vi "PLC.WriteValues.vi"(8 "error in":errorcluster, 10 "Slot":i32, 11 "Data_in":T1={"Status"={"Idx"=0, "ConnRef"=0, "State"=enum."Off", "LiveBitTimer"=timestamp(0 s since 1904-01-01)}, "Sets"={"Enable"=FALSE, "IP"="", "Rack"=0, "Slot"=0, "LifeBitTimer_s"=0.0, "DataBlockAddr_PCStatus"=0, "DataBlockAddr_PLCStatus"=1, "DataBlockAddr_PLCNewData"=[], "DataBlockSize_PLCNewData"=[], "DataBlockAddr_PLCChangeOver"=[], "DataBlockSize_PLCChangeOver"=[], "DataBlockAddr_PCChangeOver"=[], "DataBlockAddr_PLCCheckStatus"=[], "DataBlockSize_PLCCheckStatus"=[], "DataBlockAddr_PCCheckStatus"=[]}, "PCstatus"={"General"={"LifeBit"=FALSE, "DbRun"=FALSE}, "Stations"=[]}, "PLCstatus"={"General"={"LifeBit"=FALSE}, "Stations"=[]}}) -> (0 "error out":errorcluster, 3 "Data_out":T1={"Status"={"Idx"=0, "ConnRef"=0, "State"=enum."Off", "LiveBitTimer"=timestamp(0 s since 1904-01-01)}, "Sets"={"Enable"=FALSE, "IP"="", "Rack"=0, "Slot"=0, "LifeBitTimer_s"=0.0, "DataBlockAddr_PCStatus"=0, "DataBlockAddr_PLCStatus"=1, "DataBlockAddr_PLCNewData"=[], "DataBlockSize_PLCNewData"=[], "DataBlockAddr_PLCChangeOver"=[], "DataBlockSize_PLCChangeOver"=[], "DataBlockAddr_PCChangeOver"=[], "DataBlockAddr_PLCCheckStatus"=[], "DataBlockSize_PLCCheckStatus"=[], "DataBlockAddr_PCCheckStatus"=[]}, "PCstatus"={"General"={"LifeBit"=FALSE, "DbRun"=FALSE}, "Stations"=[]}, "PLCstatus"={"General"={"LifeBit"=FALSE}, "Stations"=[]}})   [LabVIEW 2016]
doc: "Get test results (measurement values) from PLC and save to database\n\nWabco 2017 All right reserved\nAuthor: maciej.szupienko@wabco-auto.com"
uses:
  LowLevel/PLC.DataBlock.PLCvalues.ctl
  PLC.Data.Sets.ctl
  PLC.State.ctl
  PLC.Data.Status.ctl
  PLC.Data.ctl
  LowLevel/PLC.DataBlock.PCstatus.ctl
  LowLevel/PLC.DataBlock.PLCstatus.ctl
  LowLevel/PLC.DataBlock.PLCstatus.Station.ctl
  LowLevel/PLC.DataBlock.PLCstatus.General.ctl
  LowLevel/PLC.DataBlock.PCstatus.Station.ctl
  LowLevel/PLC.DataBlock.PCstatus.General.ctl
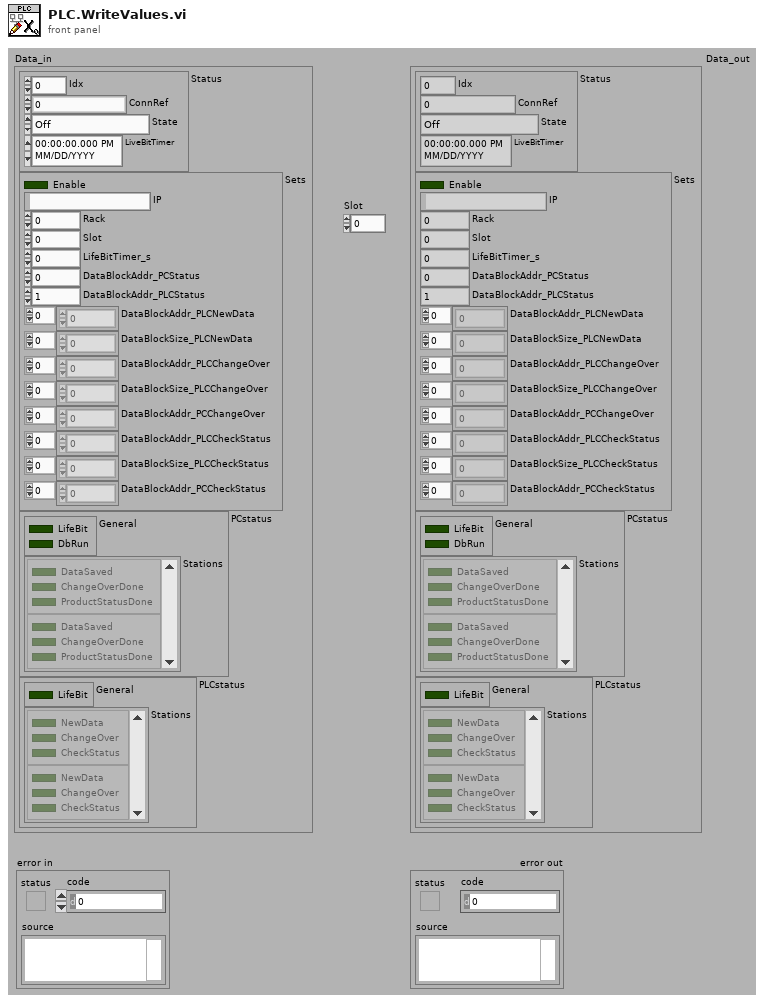
[diagram p1: front panel]
types:
  T1 = typedef "PLC.Data.ctl" = cluster{"Status":T2, "Sets":T4, "PCstatus":T5, "PLCstatus":T8}
  T2 = typedef "PLC.Data.Status.ctl" = cluster{"Idx":i32, "ConnRef":u64, "State":T3, "LiveBitTimer":timestamp}
  T3 = typedef "PLC.State.ctl" = enum32{"Off", "Error", "Idle", "Run"}
  T4 = typedef "PLC.Data.Sets.ctl" = cluster{"Enable":bool, "IP":string, "Rack":i32, "Slot":i32, "LifeBitTimer_s":dbl, "DataBlockAddr_PCStatus":i32, "DataBlockAddr_PLCStatus":i32, "DataBlockAddr_PLCNewData":i32[], "DataBlockSize_PLCNewData":i32[], "DataBlockAddr_PLCChangeOver":i32[], "DataBlockSize_PLCChangeOver":i32[], "DataBlockAddr_PCChangeOver":i32[], "DataBlockAddr_PLCCheckStatus":i32[], "DataBlockSize_PLCCheckStatus":i32[], "DataBlockAddr_PCCheckStatus":i32[]}
  T5 = typedef "PLC.DataBlock.PCstatus.ctl" = cluster{"General":T6, "Stations":T7[]}
  T6 = typedef "PLC.DataBlock.PCstatus.General.ctl" = cluster{"LifeBit":bool, "DbRun":bool}
  T7 = typedef "PLC.DataBlock.PCstatus.Station.ctl" = cluster{"DataSaved":bool, "ChangeOverDone":bool, "ProductStatusDone":bool}
  T8 = typedef "PLC.DataBlock.PLCstatus.ctl" = cluster{"General":T9, "Stations":T10[]}
  T9 = typedef "PLC.DataBlock.PLCstatus.General.ctl" = cluster{"LifeBit":bool}
  T10 = typedef "PLC.DataBlock.PLCstatus.Station.ctl" = cluster{"NewData":bool, "ChangeOver":bool, "CheckStatus":bool}
  T11 = typedef "PLC.DataBlock.PLCvalues.ctl" = cluster{"Status":u8, "Ref1":string, "Serial1":string, "Ref2":string, "Serial2":string, "Values":sgl[]}
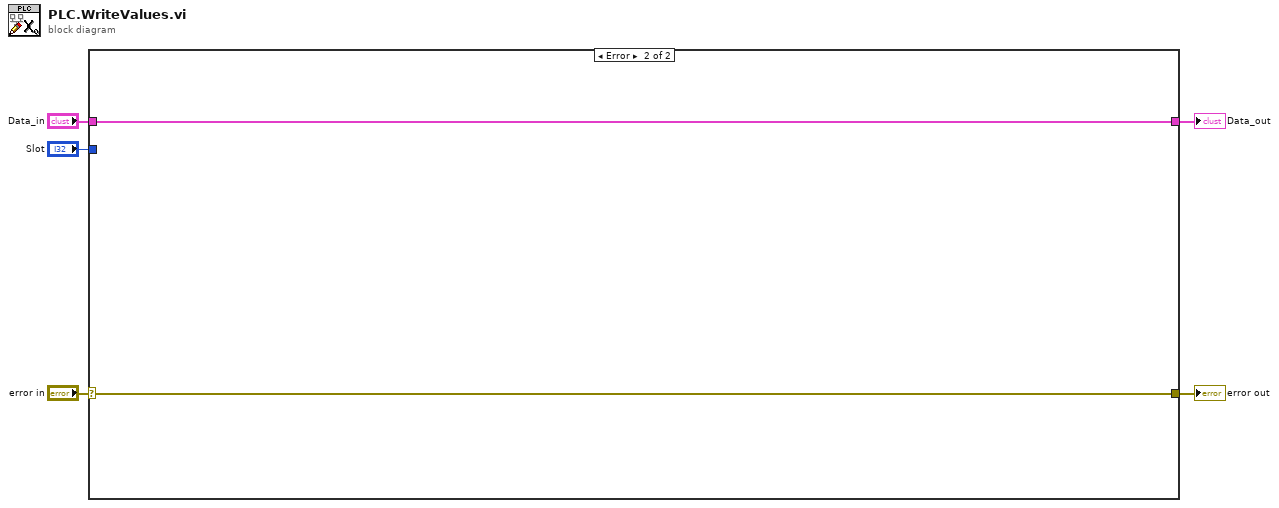
[diagram p0: block diagram]
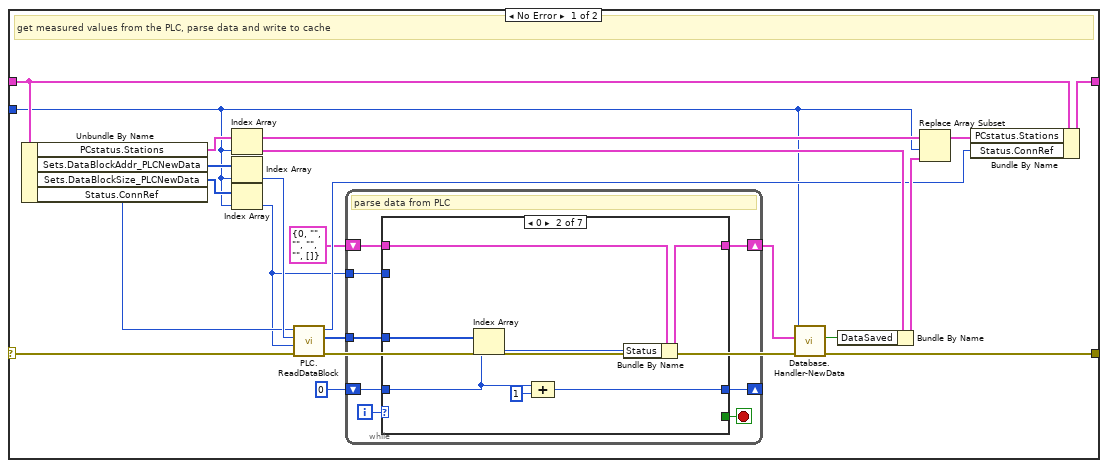
[diagram p2: hidden frame]
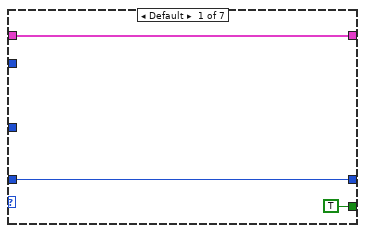
[diagram p3: hidden frame]
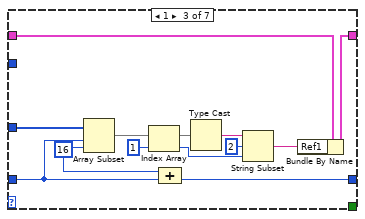
[diagram p4: hidden frame]
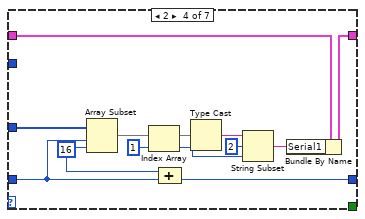
[diagram p5: hidden frame]
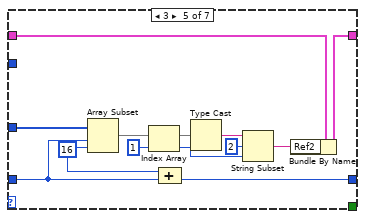
[diagram p6: hidden frame]
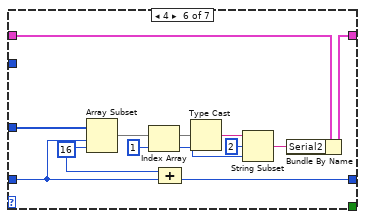
[diagram p7: hidden frame]
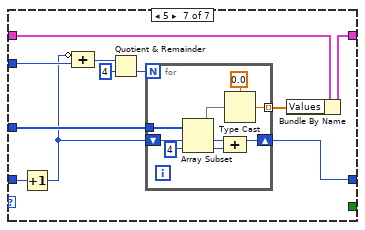
[diagram p8: hidden frame]
diagram:
  n1 = case shown="Error" "error in" {
    selector: "error in" -> [w25 w112]
    tunnel: [w6 w112] -> w2
    tunnel: "Data_in" -> [w22 w111]
    tunnel: [w26 w111] -> w4
    tunnel: "Slot" -> [w10 _]
    frame No Error {
      # "get measured values from the PLC, parse data and write to cache"
      n2 = Unbundle By Name(w22) -> ("PCstatus.Stations"=w12:T7[], "Sets.DataBlockAddr_PLCNewData"=w24:i32[], "Sets.DataBlockSize_PLCNewData"=w11:i32[], "Status.ConnRef"=w21:u64)
      n3 = Index Array(array=w12, index=w10) -> (element=w19:T7)
      n4 = Index Array(array=w24, index=w10) -> (element=w23:i32)
      n5 = Index Array(array=w11, index=w10) -> (element=w13:i32)
      n6 = call "PLC.ReadDataBlock.vi"("error in (no error)"=w25, "Amount (1)"=w13, "Block"=w23, "Ref"=w21) -> ("error out"=w8:errorcluster, "data out"=w16:u8[], "ref out"=w17:u64)  [unwired: 5 in]
      n7 = while {
        tunnel: w16 -> [w29]
        shift-right: [w32] -> _
        shift-left: 0 -> [w33]
        shift-right: [w31] -> w9
        shift-left: T11 {"Status"=0, "Ref1"="", "Serial1"="", "Ref2"="", "Serial2"="", "Values"=[]} ("element") -> [w30]
        tunnel: w13 -> [w28]
        i -> [w34]
        stop <- w27 stop-if-true
        # "parse data from PLC"
        n8 = case shown="0" w34 {
          tunnel: w33 -> [w36 w41 w47 w59 w71 w83 w94]
          tunnel: [w36 w42 w46 w58 w70 w82 w97] -> w32
          tunnel: [w37 w40 w56 w68 w80 w92 w102] -> w31
          tunnel: w30 -> [w37 w39 w55 w67 w79 w91 w103]
          tunnel: w29 -> [_ w44 w50 w62 w74 w86 w98]
          tunnel: w28 -> [_ _ _ _ _ _ w96]
          tunnel: [TRUE _ _ _ _ _ _] -> w27
          frame Default {
          }
          frame 0 {
            n9 = Index Array(array=w44, index=w41) -> (element=w43:u8)
            n10 = Compound Arithmetic op=ADD(w41, 1 ("value")) -> (w42:i32)
            n11 = Bundle By Name(cluster=w39, "Status"=w43) -> (w40:T11)
          }
          frame 1 {
            w48 = 16 ("length")
            n12 = Array Subset(array=w50, index=w47, length=w48) -> (w52:u8[])
            n13 = Index Array(array=w52, index=1) -> (element=w45:u8)
            n14 = Compound Arithmetic op=ADD(w48, w47) -> (w46:i32)
            n15 = Type Cast(x=w52) -> (*(type *) &x=w51:string)  [unwired: 1 in]
            n16 = String Subset(string=w51, offset (0)=2, length (rest)=w45) -> (substring=w49:string)
            n17 = Bundle By Name(cluster=w55, "Ref1"=w49) -> (w56:T11)
          }
          frame 2 {
            w60 = 16 ("length")
            n18 = Array Subset(array=w62, index=w59, length=w60) -> (w64:u8[])
            n19 = Index Array(array=w64, index=1) -> (element=w57:u8)
            n20 = Compound Arithmetic op=ADD(w60, w59) -> (w58:i32)
            n21 = Type Cast(x=w64) -> (*(type *) &x=w63:string)  [unwired: 1 in]
            n22 = String Subset(string=w63, offset (0)=2, length (rest)=w57) -> (substring=w61:string)
            n23 = Bundle By Name(cluster=w67, "Serial1"=w61) -> (w68:T11)
          }
          frame 3 {
            w72 = 16 ("length")
            n24 = Array Subset(array=w74, index=w71, length=w72) -> (w76:u8[])
            n25 = Index Array(array=w76, index=1) -> (element=w69:u8)
            n26 = Compound Arithmetic op=ADD(w72, w71) -> (w70:i32)
            n27 = Type Cast(x=w76) -> (*(type *) &x=w75:string)  [unwired: 1 in]
            n28 = String Subset(string=w75, offset (0)=2, length (rest)=w69) -> (substring=w73:string)
            n29 = Bundle By Name(cluster=w79, "Ref2"=w73) -> (w80:T11)
          }
          frame 4 {
            w84 = 16 ("length")
            n30 = Array Subset(array=w86, index=w83, length=w84) -> (w88:u8[])
            n31 = Index Array(array=w88, index=1) -> (element=w81:u8)
            n32 = Compound Arithmetic op=ADD(w84, w83) -> (w82:i32)
            n33 = Type Cast(x=w88) -> (*(type *) &x=w87:string)  [unwired: 1 in]
            n34 = String Subset(string=w87, offset (0)=2, length (rest)=w81) -> (substring=w85:string)
            n35 = Bundle By Name(cluster=w91, "Serial2"=w85) -> (w92:T11)
          }
          frame 5 {
            n36 = Increment(x=w94) -> (x+1=w93:i32)
            n37 = Compound Arithmetic op=ADD(invert w93, w96) -> (w101:i32)
            n38 = Quotient & Remainder(x=w101, y=4) -> (floor(x/y)=w95:i32)  [unwired: 1 out]
            n39 = for {
              N: w95 -> [_]
              shift-right: [w108] -> w97
              shift-left: w93 -> [w109]
              tunnel: w98 -> [w110]
              tunnel: [w105] -> w99 mode=indexing
              w107 = 4 ("length")
              n40 = Array Subset(array=w110, index=w109, length=w107) -> (w106:u8[])
              n41 = Compound Arithmetic op=ADD(w109, w107) -> (w108:i32)
              n42 = Type Cast(type=sgl 0.0 ("index"), x=w106) -> (*(type *) &x=w105:sgl)
            }
            n43 = Bundle By Name(cluster=w103, "Values"=w99) -> (w102:T11)
          }
        }
      }
      n44 = call "Database.Handler-NewData.vi"("error in"=w8, "Data"=w9, "Idx"=w10) -> ("error out"=w6:errorcluster, "Saved"=w7:bool)  [unwired: 7 in]
      n45 = Bundle By Name(cluster=w19, "DataSaved"=w7) -> (w18:T7)
      n46 = Replace Array Subset(array=w12, new element=w18, index=w10) -> (w20:T7[])
      n47 = Bundle By Name(cluster=w22, "PCstatus.Stations"=w20, "Status.ConnRef"=w17) -> (w26:T1)
    }
    frame Error {
    }
  }
  "error out" <- w2
  "Data_out" <- w4
